vi "Unpack For Grpc.vi"(8 "error in (no error)":errorcluster, 9 "Configuration / Resuls (Config)":enum16{"Configuration", "Results"}(ring), 10 "Any":T1, 11 "Measurement Customizations in":refnum<class "Measurement Plugin.lvclass">) -> (0 "error out":errorcluster, 2 "Data Value":variant, 3 "Measurement Customizations out":refnum<class "Measurement Plugin.lvclass">)   [LabVIEW 2020, in "NIScopeAcquireWaveform.lvlib" / "Measurement Plugin.lvclass"]
uses:
  Measurement Plugin.lvclass
  <vilib>/gRPC/LabVIEW gRPC Library/Shared/Any.ctl
  Measurement Configuration.ctl
  <instrlib>/niScope/Controls/niScope vertical coupling.ctl
  <instrlib>/niScope/Controls/niScope trigger slope.ctl
  Measurement Results.ctl
  a521b266-ce99-437c-923d-067dcf1e07fd.vi
  3ecd018e-d556-4cbc-bc60-c4ba57204520.vi
  <vilib>/gRPC/LabVIEW gRPC Library/Server API/Translate Protobuf Error.vi
  <vilib>/AdvancedString/1D String Array to Delimited String.vi
  <vilib>/gRPC/LabVIEW gRPC Library/Server API/Server/Get Server DLL Path.vi
  NIScopeAcquireWaveform.lvlib
  <vilib>/gRPC/LabVIEW gRPC Library/grpc-lvsupport-release.lvlib
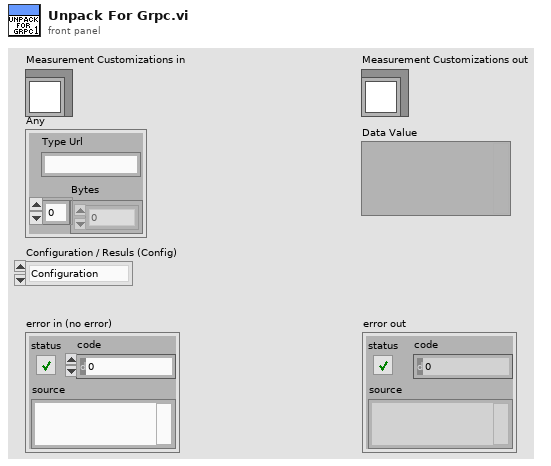
[diagram p1: front panel]
types:
  T1 = typedef "grpc-lvsupport-release.lvlib/Any.ctl" = cluster{"Type Url":string, "Bytes":u8[]}
  T2 = typedef "grpc-lvsupport-release.lvlib/grpcId.ctl" = u64
  T3 = typedef "NIScopeAcquireWaveform.lvlib/Measurement Configuration.ctl" = cluster{"Pin Names":string[], "Vertical Range":dbl, "Vertical Coupling":T4, "Input Impedance":u32, "Minimum Sample Rate":dbl, "Minimum Record Length":i32, "Trigger Source":string, "Trigger Level":dbl, "Trigger Slope":T5, "Timeout":dbl, "Trigger Coupling":u32}
  T4 = typedef "niScope vertical coupling.ctl" = i32
  T5 = typedef "niScope trigger slope.ctl" = i32
  T6 = typedef "NIScopeAcquireWaveform.lvlib/Measurement Results.ctl" = cluster{"Waveform0":dbl[], "Waveform1":dbl[], "Waveform2":dbl[], "Waveform3":dbl[]}
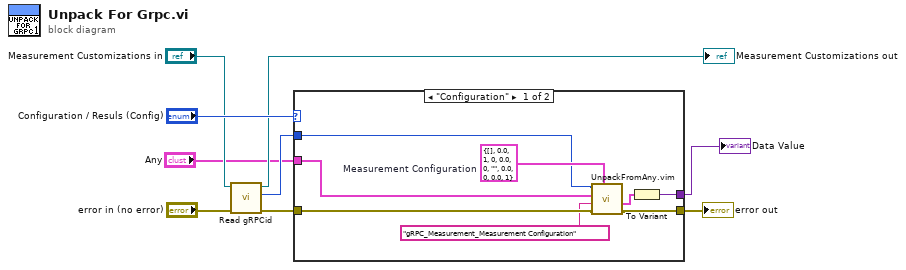
[diagram p0: block diagram]
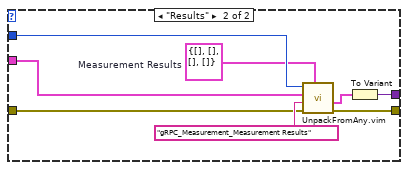
[diagram p2: hidden frame]
diagram:
  n1 = call-dynamic "Read gRPCid.vi"("error in (no error)"="error in (no error)", "MeasurementPluginService in"="Measurement Customizations in") -> ("error out"=w6:errorcluster, "gRPCid"=w3:T2, "MeasurementPluginService out"=→"Measurement Customizations out":refnum<class "Measurement Plugin.lvclass">)  [unwired: 7 in]
  n2 = case shown="\"Configuration\"" "Configuration / Resuls (Config)" {
    tunnel: w6 -> [w15 w19]
    tunnel: "Any" -> [w10 w18]
    tunnel: w3 -> [w12 w22]
    tunnel: [w16 w23] -> w9
    tunnel: [w17 w25] -> w1
    frame "Configuration" {
      w13 = T3 {"Pin Names"=[], "Vertical Range"=0.0, "Vertical Coupling"=1, "Input Impedance"=0, "Minimum Sample Rate"=0.0, "Minimum Record Length"=0, "Trigger Source"="", "Trigger Level"=0.0, "Trigger Slope"=0, "Timeout"=0.0, "Trigger Coupling"=1}  # Measurement Configuration
      n3 = call "UnpackFromAny.vim"("Data Type"=w13, "error in"=w15, "Message Type"="gRPC_Measurement_Measurement Configuration", "Any"=w10, "gRPCid in"=w12) -> ("error out"=w16:errorcluster, "Unpacked Value"=w14:T3)  [unwired: 4 in, 1 out]
      n4 = To Variant(anything=w14) -> (Variant=w17:variant)
    }
    frame "Results" {
      w21 = T6 {"Waveform0"=[], "Waveform1"=[], "Waveform2"=[], "Waveform3"=[]}  # Measurement Results
      n5 = call "UnpackFromAny.vim"("Data Type"=w21, "error in"=w19, "Message Type"="gRPC_Measurement_Measurement Results", "Any"=w18, "gRPCid in"=w22) -> ("error out"=w23:errorcluster, "Unpacked Value"=w24:T6)  [unwired: 4 in, 1 out]
      n6 = To Variant(anything=w24) -> (Variant=w25:variant)
    }
  }
  "error out" <- w9
  "Data Value" <- w1
